vi "Bin Logging Message Loop.vi"(8 "error in (no error)":errorcluster, 10 "Data Queue":refnum<queue>, 11 "Message Queues":T1) -> (0 "error out":errorcluster)   [LabVIEW 2017, in "Logging.lvlib"]
uses:
  Logging.lvlib
  support/Message Queue/All Message Queues.ctl
  support/Message Queue/Message Cluster.ctl
  Logging Configuration.ctl
  Logging State.ctl
  support/Message Queue/Enqueue Message (Single).vi
  <vilib>/Utility/error.llb/Error Cluster From Error Code.vi
  <vilib>/ErrorRing/Error Ring.xnode
  support/Message Queue/Message Queue.lvlib
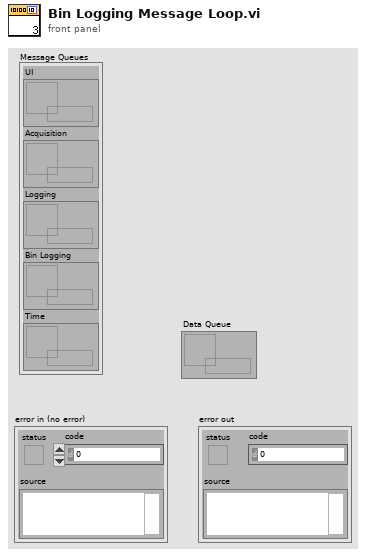
[diagram p1: front panel]
types:
  T1 = typedef "Message Queue.lvlib/All Message Queues.ctl" = cluster{"UI":refnum<queue>, "Acquisition":refnum<queue>, "Logging":refnum<queue>, "Bin Logging":refnum<queue>, "Time":refnum<queue>}
  T2 = typedef "Logging.lvlib/Logging Configuration.ctl" = cluster{"Log File Base Path":path, "TDMS File Reference":refnum<k34>, "Log File Offsite Path":path, "Project code":string, "Bin File Reference":refnum<file>}
  T3 = enum16{"open", "replace", "create", "open or create", "replace or create", "replace or create with confirmation"}
  T4 = typedef "Logging.lvlib/Logging State.ctl" = enum16{"Idle", "Logging"}
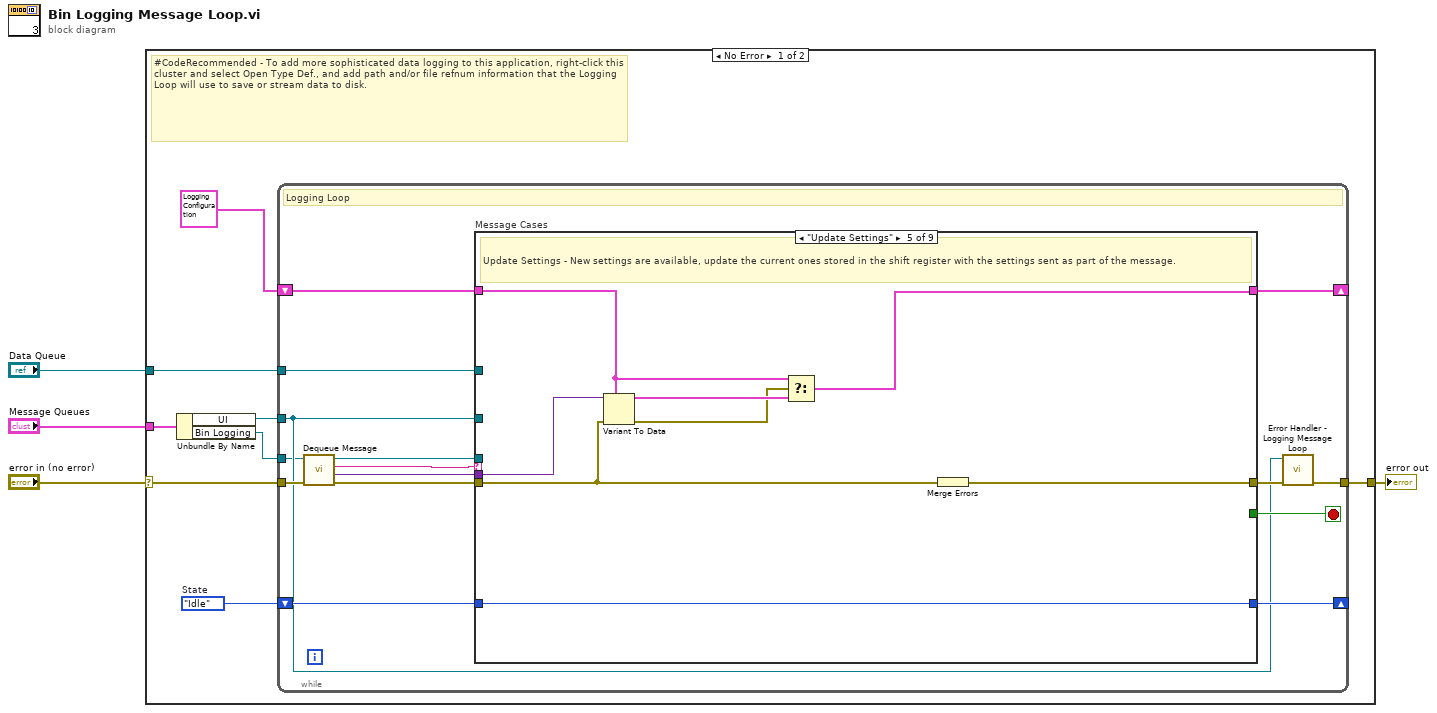
[diagram p0: block diagram]
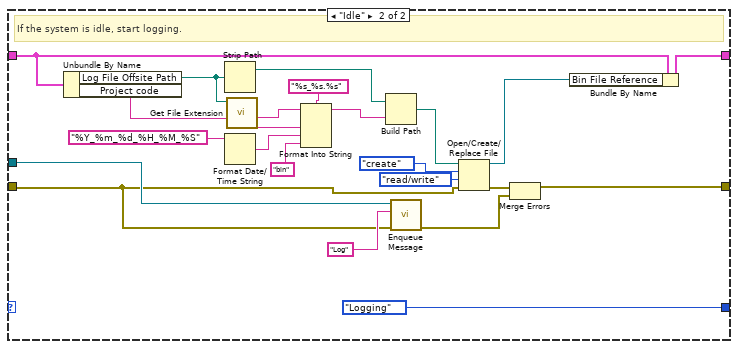
[diagram p4: hidden frame]
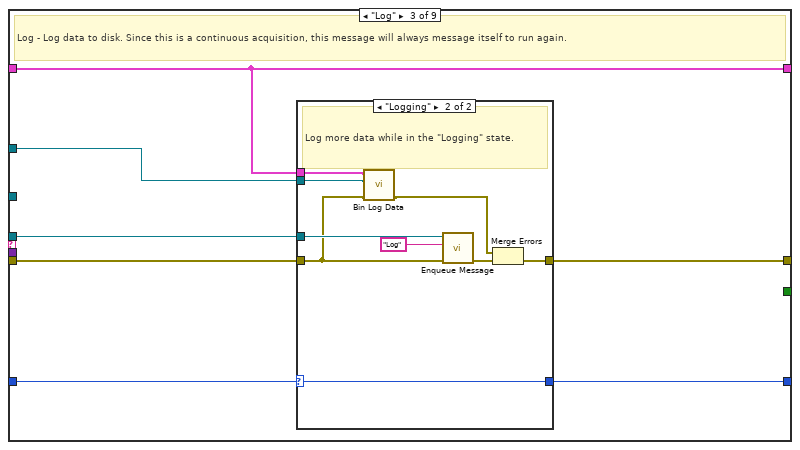
[diagram p5: hidden frame]
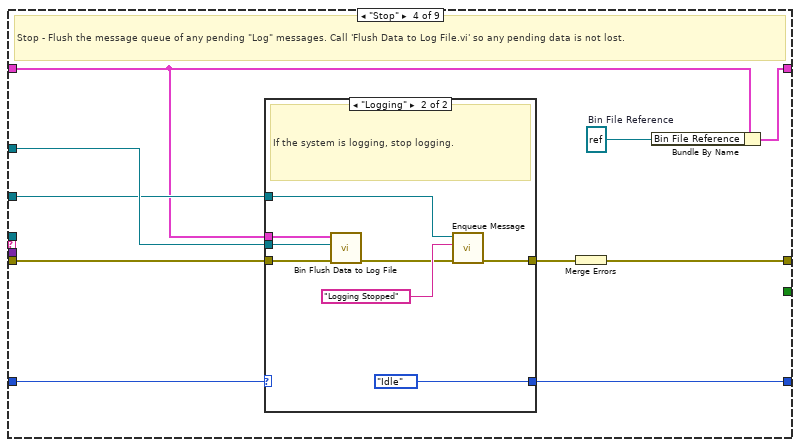
[diagram p7: hidden frame]
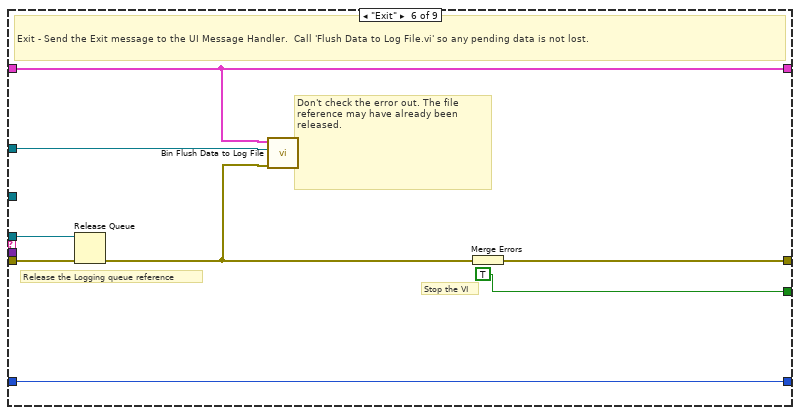
[diagram p9: hidden frame]
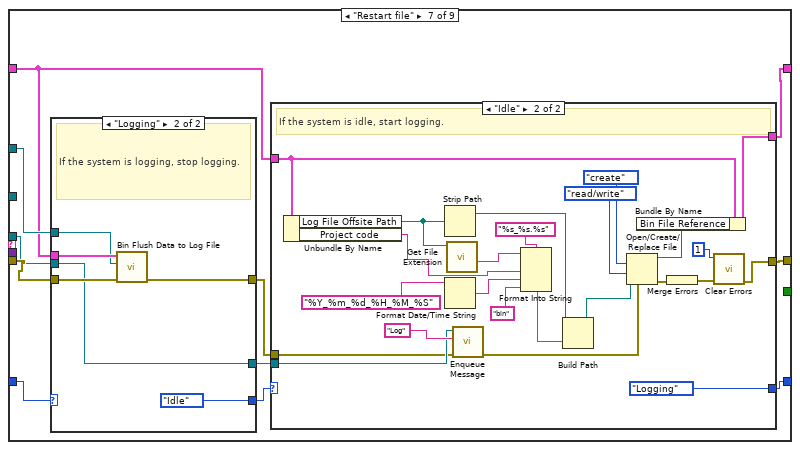
[diagram p10: hidden frame]
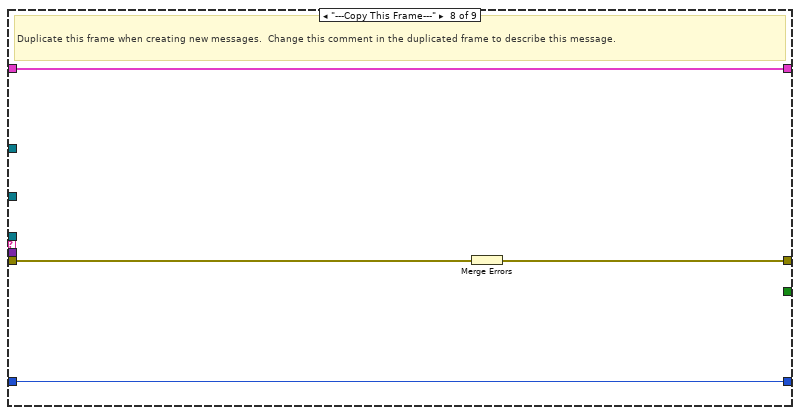
[diagram p13: hidden frame]
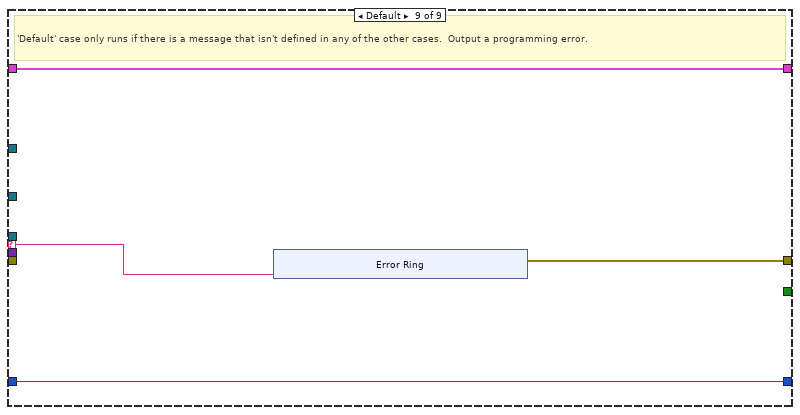
[diagram p14: hidden frame]
diagram:
  n1 = case shown="No Error" "error in (no error)" {
    selector: "error in (no error)" -> [w9 w178]
    tunnel: "Message Queues" -> [w12 _]
    tunnel: [w11 w178] -> w3
    tunnel: "Data Queue" -> [w8 _]
    frame No Error {
      w6 = Logging_State."Idle"  # State
      # "#CodeRecommended - To add more sophisticated data logging to this application, right-click this cluster and select Open Type Def., and add path and/or file refnum information that the Logging Loop will use to save or stream data to disk."
      n2 = Unbundle By Name(w12) -> ("UI"=w7:refnum<queue>, "Bin Logging"=w5:refnum<queue>)
      n3 = while {
        shift-right: [w27] -> _
        shift-left: T2 {"Log File Base Path"=path "", "TDMS File Reference"=refnum, "Log File Offsite Path"=path "", "Project code"="", "Bin File Reference"=refnum} ("Logging Configuration") -> [w14]
        tunnel: w7 -> [w16]
        tunnel: w8 -> [w21]
        shift-right: [w19] -> _
        shift-left: w6 -> [w20]
        tunnel: w9 -> [w25]
        tunnel: [w18] -> w11
        tunnel: w5 -> [w15]
        stop <- w26 stop-if-true
        # "Logging Loop"
        n4 = call "Dequeue Message.vi"("error in (no error)"=w25, "Message Queue"=w15) -> ("error out"=w24:errorcluster, "Message Data"=w23:variant, "Message"=w13:string, "dup Message Queue"=w22:refnum<queue>)  [unwired: 6 in]
        n5 = case "Message Cases" shown="\"Update Settings\"" w13 {
          selector: w13 -> [_ _ _ _ _ _ _ _ w167]
          tunnel: w22 -> [_ w36 w68 _ _ w113 w126 _ _]
          tunnel: w24 -> [w29 w35 w66 w87 w101 w114 w127 w166 _]
          tunnel: [w29 w37 w69 w90 w108 w115 w122 w164 w168] -> w17
          tunnel: w14 -> [w30 w34 w65 w83 w107 w111 w117 w165 w170]
          tunnel: [w30 w33 w65 w82 w104 w111 w121 w165 w170] -> w27
          tunnel: [_ _ _ _ _ TRUE _ _ _] -> w26
          tunnel: w23 -> [_ _ _ _ w102 _ _ _ _]
          tunnel: w16 -> [_ _ _ w84 _ _ _ _ _]
          tunnel: w21 -> [_ _ w67 w88 _ w109 w119 _ _]
          tunnel: w20 -> [w28 w32 w64 w86 w103 w112 w120 w163 w169]
          tunnel: [w28 w31 w63 w85 w103 w112 w123 w163 w169] -> w19
          frame "Initialize" {
            # "Initialize - gets called when first launched. Currently a no-op."
          }
          frame "Start" {
            # "Start - Send the \"Log\" message to start logging.  Generate a unique, timestamped TDMS file name based on the Log File Base Path value."
            n6 = case shown="\"Logging\"" w32 {
              selector: w32 -> [w39 _]
              tunnel: [w38 w48] -> w37
              tunnel: w36 -> [_ w49]
              tunnel: w35 -> [w38 w42]
              tunnel: w34 -> [w40 w50]
              tunnel: [w40 w52] -> w33
              tunnel: [w39 Logging_State."Logging" ("State")] -> w31
              frame "Logging" {
                # "The system is already logging. Ignore the \"Start\" message."
              }
              frame "Idle" {
                # "If the system is idle, start logging."
                n7 = Unbundle By Name(w50) -> ("Log File Offsite Path"=w61:path, "Project code"=w47:string)
                n8 = Strip Path(path=w61) -> (stripped path=w58:path)  [unwired: 1 out]
                n9 = Format Date/Time String(time format string (%c)="%Y_%m_%d_%H_%M_%S") -> (date/time string=w56:string)  [unwired: 2 in]
                n10 = call <vilib>:"Get File Extension.vi"("file"=w61) -> ("filename without extension"=w59:string)  [unwired: 6 in, 4 out]
                n11 = Format Into String(format string="%s_%s.%s", initial string=w59, w47, w56, "bin" ("input 3")) -> (resulting string=w54:string)  [unwired: 1 in, 1 out]
                n12 = Build Path(base path=w58, name or relative path=w54) -> (appended path=w45:path)
                n13 = call-poly "Enqueue Message.vi"("error in (no error)"=w42, "Message"="Log", "Message Queue"=w49) -> ("error out"=w53:errorcluster)  [unwired: 7 in, 1 out]
                n14 = Open/Create/Replace File(file path (use dialog)=w45, error in=w42, operation (0:open)=T3."create", access (0:read/write)=enum16{"read/write", "read-only", "write-only"}."read/write") -> (refnum out=w41:refnum<file>, error out=w46:errorcluster)  [unwired: 2 in, 1 out]
                n15 = Merge Errors(w46, w53) -> (w48:errorcluster)
                n16 = Bundle By Name(cluster=w50, "Bin File Reference"=w41) -> (w52:T2)
              }
            }
          }
          frame "Log" {
            # "Log - Log data to disk. Since this is a continuous acquisition, this message will always message itself to run again."
            n17 = case shown="\"Logging\"" w64 {
              selector: w64 -> [w71 w76]
              tunnel: [w70 w80] -> w69
              tunnel: w68 -> [_ w78]
              tunnel: w67 -> [_ w74]
              tunnel: w66 -> [w70 w73]
              tunnel: w65 -> [_ w75]
              tunnel: [w71 w76] -> w63
              frame "Idle" {
                # "Ignore \"Log\" messages when the logging is idle."
              }
              frame "Logging" {
                # "Log more data while in the \"Logging\" state."
                n18 = call "Bin Log Data.vi"("error in (no error)"=w73, "Data Queue"=w74, "Logging Configuration"=w75) -> ("error out"=w72:errorcluster)  [unwired: 8 in]
                n19 = call-poly "Enqueue Message.vi"("error in (no error)"=w73, "Message"="Log", "Message Queue"=w78) -> ("error out"=w79:errorcluster)  [unwired: 7 in, 1 out]
                n20 = Merge Errors(w72, w79) -> (w80:errorcluster)
              }
            }
          }
          frame "Stop" {
            w81 = refnum<file> refnum  # Bin File Reference
            # "Stop - Flush the message queue of any pending \"Log\" messages. Call 'Flush Data to Log File.vi' so any pending data is not lost."
            n21 = case shown="\"Logging\"" w86 {
              selector: w86 -> [w91 _]
              tunnel: [w92 w99] -> w89
              tunnel: w88 -> [_ w95]
              tunnel: w83 -> [_ w96]
              tunnel: w87 -> [w92 w94]
              tunnel: [w91 Logging_State."Idle" ("State")] -> w85
              tunnel: w84 -> [_ w98]
              frame "Idle" {
                # "The system is already idle. Ignore the \"Stop\" message."
              }
              frame "Logging" {
                # "If the system is logging, stop logging."
                n22 = call "Bin Flush Data to Log File.vi"("error in (no error)"=w94, "Data Queue"=w95, "Logging Configuration"=w96) -> ("error out"=w93:errorcluster)  [unwired: 8 in]
                n23 = call-poly "Enqueue Message.vi"("error in (no error)"=w93, "Message"="Logging Stopped", "Message Queue"=w98) -> ("error out"=w99:errorcluster)  [unwired: 7 in, 1 out]
              }
            }
            n24 = Merge Errors(w89) -> (w90:errorcluster)
            n25 = Bundle By Name(cluster=w83, "Bin File Reference"=w81) -> (w82:T2)
          }
          frame "Update Settings" {
            # "Update Settings - New settings are available, update the current ones stored in the shift register with the settings sent as part of the message."
            n26 = Variant To Data(error in=w101, type=w107, Variant=w102) -> (data=w106:T2, error out=w105:errorcluster)
            n27 = Select(t=w107, s=w105, f=w106) -> (s? t:f=w104:T2)
            n28 = Merge Errors(w101) -> (w108:errorcluster)
          }
          frame "Exit" {
            # "Don't check the error out. The file reference may have already been released."
            # "Release the Logging queue reference"
            # "Stop the VI"
            # "Exit - Send the Exit message to the UI Message Handler.  Call 'Flush Data to Log File.vi' so any pending data is not lost."
            n29 = Release Queue(queue=w113, error in (no error)=w114) -> (error out=w110:errorcluster)  [unwired: 1 in, 2 out]
            n30 = call "Bin Flush Data to Log File.vi"("error in (no error)"=w110, "Data Queue"=w109, "Logging Configuration"=w111) -> ()  [unwired: 8 in, 1 out]
            n31 = Merge Errors(w110) -> (w115:errorcluster)
          }
          frame "Restart file" {
            n32 = case shown="\"Logging\"" w120 {
              selector: w120 -> [w155 _]
              tunnel: [w156 w159] -> w125
              tunnel: w126 -> [_ w157]
              tunnel: w117 -> [_ w161]
              tunnel: w127 -> [w156 w160]
              tunnel: [w155 Logging_State."Idle" ("State")] -> w124
              tunnel: w119 -> [_ w158]
              tunnel: [_ w157] -> w118
              frame "Idle" {
                # "The system is already idle. Ignore the \"Stop\" message."
              }
              frame "Logging" {
                # "If the system is logging, stop logging."
                n33 = call "Bin Flush Data to Log File.vi"("error in (no error)"=w160, "Data Queue"=w158, "Logging Configuration"=w161) -> ("error out"=w159:errorcluster)  [unwired: 8 in]
              }
            }
            n34 = case shown="\"Idle\"" w124 {
              selector: w124 -> [w130 _]
              tunnel: [w129 w131] -> w122
              tunnel: [w128 w147] -> w121
              tunnel: [w130 Logging_State."Logging" ("State")] -> w123
              tunnel: w117 -> [w128 w138]
              tunnel: w125 -> [w129 w135]
              tunnel: w118 -> [_ w136]
              frame "Logging" {
                # "The system is already logging. Ignore the \"Start\" message."
              }
              frame "Idle" {
                # "If the system is idle, start logging."
                n35 = Unbundle By Name(w138) -> ("Log File Offsite Path"=w140:path, "Project code"=w139:string)
                n36 = Strip Path(path=w140) -> (stripped path=w152:path)  [unwired: 1 out]
                n37 = Format Date/Time String(time format string (%c)="%Y_%m_%d_%H_%M_%S") -> (date/time string=w150:string)  [unwired: 2 in]
                n38 = call <vilib>:"Get File Extension.vi"("file"=w140) -> ("filename without extension"=w153:string)  [unwired: 6 in, 4 out]
                n39 = call-poly "Enqueue Message.vi"("error in (no error)"=w135, "Message"="Log", "Message Queue"=w136) -> ("error out"=w134:errorcluster)  [unwired: 7 in, 1 out]
                n40 = Format Into String(format string="%s_%s.%s", initial string=w153, w139, w150, "bin" ("input 3")) -> (resulting string=w148:string)  [unwired: 1 in, 1 out]
                n41 = Build Path(base path=w152, name or relative path=w148) -> (appended path=w144:path)
                n42 = Open/Create/Replace File(file path (use dialog)=w144, error in=w134, operation (0:open)=T3."create", access (0:read/write)=enum16{"read/write", "read-only", "write-only"}."read/write") -> (refnum out=w141:refnum<file>, error out=w145:errorcluster)  [unwired: 2 in, 1 out]
                n43 = Bundle By Name(cluster=w138, "Bin File Reference"=w141) -> (w147:T2)
                n44 = Merge Errors(w145) -> (w133:errorcluster)
                n45 = call <vilib>:"Clear Errors.vi"("error in (no error)"=w133, "specific error code to clear (0: all)"=1) -> ("error out"=w131:errorcluster)  [unwired: 4 in, 1 out]
              }
            }
          }
          frame "---Copy This Frame---" {
            # "Duplicate this frame when creating new messages.  Change this comment in the duplicated frame to describe this message."
            n46 = Merge Errors(w166) -> (w164:errorcluster)
          }
          frame Default {
            # "'Default' case only runs if there is a message that isn't defined in any of the other cases.  Output a programming error."
            n47 = xnode "Error Ring"("parameter 0"=w167) -> ("error out"=w168:errorcluster)
          }
        }
        n48 = call "Error Handler - Logging Message Loop.vi"("error in (no error)"=w17, "Message Queue"=w16) -> ("dup error in"=w18:errorcluster)  [unwired: 8 in, 1 out]
      }
    }
    frame Error {
    }
  }
  "error out" <- w3
